vi "logarytmliniowy.vi"(1 "Liniowy/logarytmiczny":bool, 2 "Amplituda":dbl, 3 "Ilosc probek":u32, 4 "F min":dbl, 5 "F max":dbl) -> (0 "Czestotliwosc":dbl[](array[numeric]))   [LabVIEW 2021]
doc: "wybór wartoœci logarytmicznie lub liniowo dla czêstotliwoœci"
panel:
  out "Amplituda":dbl
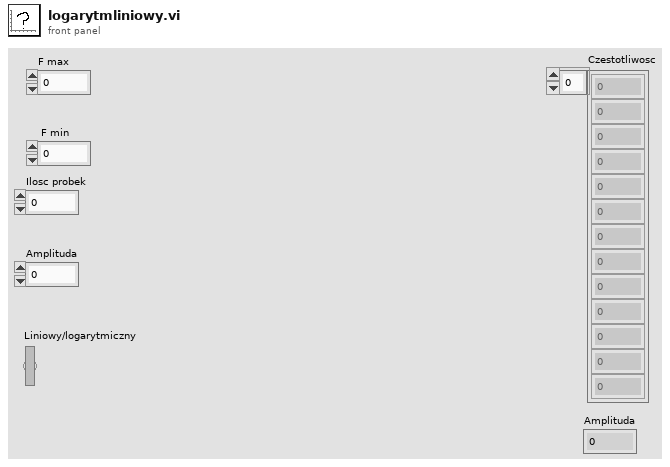
[diagram p1: front panel]
types:
  T1 = typedef "controlmaszyna.ctl" = enum16{"init", "praca", "pomiar", "wykres", "zapis", "stop", "koniec"}
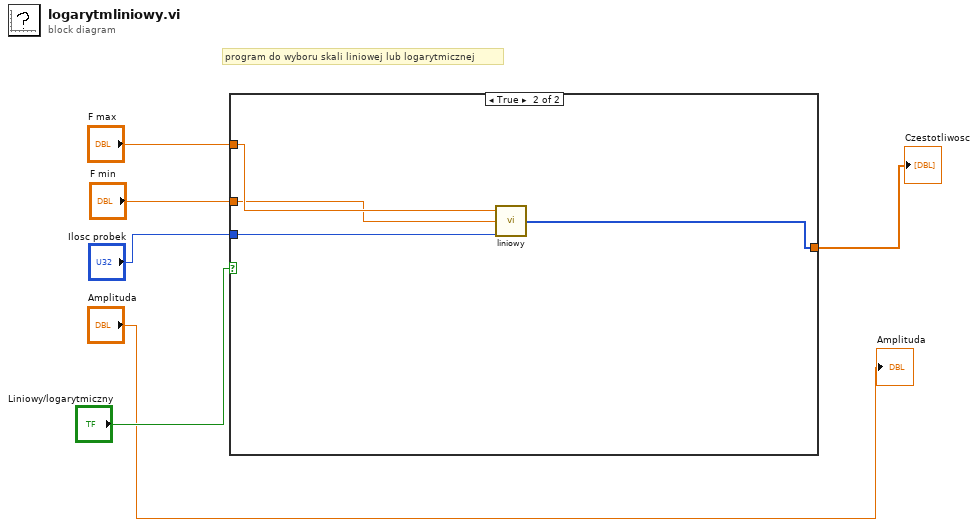
[diagram p0: block diagram]
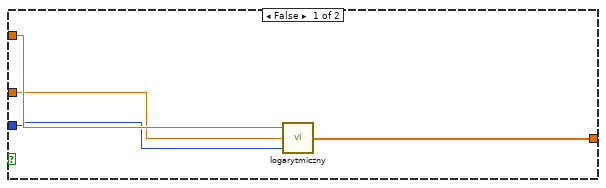
[diagram p2: hidden frame]
diagram:
  # "program do wyboru skali liniowej lub logarytmicznej"
  n1 = case shown="True" "Liniowy/logarytmiczny" {
    tunnel: "F max" -> [w10 w14]
    tunnel: "F min" -> [w9 w13]
    tunnel: "Ilosc probek" -> [w8 w12]
    tunnel: [w7 w11] -> w2
    frame False {
      n2 = call "logarytmiczny.vi"("Ilosc probek"=w8, "F min"=w9, "F max"=w10) -> ("Array"=w7:dbl[])
    }
    frame True {
      n3 = call "liniowy.vi"("ilosc probek"=w12, "F min"=w13, "F max"=w14) -> ("Tabela"=w11:T1[])
    }
  }
  "Czestotliwosc" <- w2
  "Amplituda" <- "Amplituda"
